vi "Open Device.vi"(8 "error in (no error)":errorcluster, 11 "Device":refnum<class "Device.lvclass">) -> (0 "error out":errorcluster, 3 "Device out":refnum<class "Device.lvclass">)   [LabVIEW 2015, in "Device.lvclass"]
uses:
  Device.lvclass
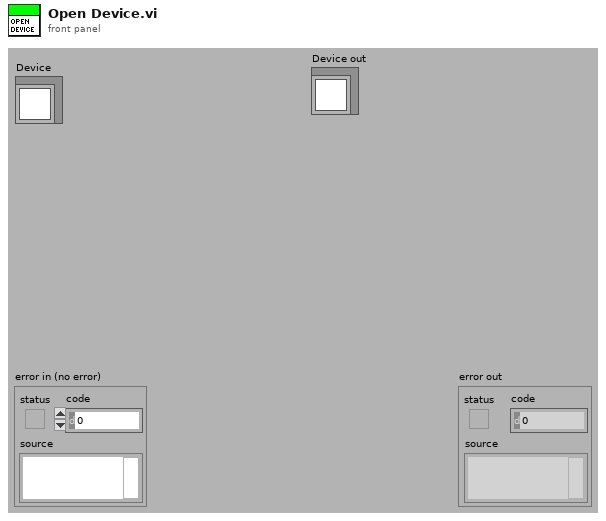
[diagram p1: front panel]
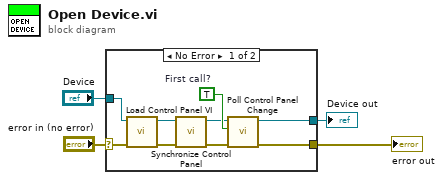
[diagram p0: block diagram]
diagram:
  n1 = case shown="No Error" "error in (no error)" {
    selector: "error in (no error)" -> [w7 w15]
    tunnel: [w6 w15] -> w1
    tunnel: [w5 w14] -> w2
    tunnel: "Device" -> [w13 w14]
    frame No Error {
      w11 = TRUE  # First call?
      n2 = call "Load Control Panel VI.vi"("error in (no error)"=w7, "Device"=w13) -> ("error out"=w9:errorcluster, "Device out"=w12:refnum<class "Device.lvclass">)  [unwired: 7 in, 1 out]
      n3 = call-dynamic "Synchronize Control Panel.vi"("error in (no error)"=w9, "Device"=w12) -> ("error out"=w8:errorcluster, "Device out"=w10:refnum<class "Device.lvclass">)  [unwired: 8 in]
      n4 = call "Poll Control Panel Change.vi"("error in (no error)"=w8, "First call?"=w11, "Device"=w10) -> ("error out"=w6:errorcluster, "Device out"=w5:refnum<class "Device.lvclass">)  [unwired: 7 in]
    }
    frame Error {
    }
  }
  "error out" <- w1
  "Device out" <- w2
